vi "Number_To_String.vi"(1 "Number":dbl) -> (0 "String":string)   [LabVIEW 2011]
doc: "This VI will convert a number to a string without appending any unecessary zeros."
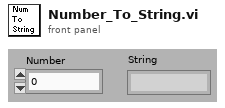
[diagram p1: front panel]
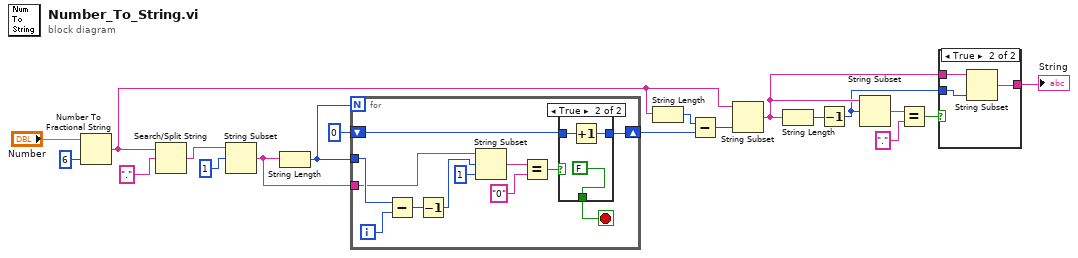
[diagram p0: block diagram]
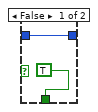
[diagram p3: hidden frame]
diagram:
  n1 = Number To Fractional String(number="Number", precision (6)=i16 6) -> (F-format string=w9:string)  [unwired: 2 out]
  n2 = Search/Split String(string=w9, search string/char (-)="." ("search string")) -> (match + rest of string=w12:string)  [unwired: 3 out]
  n3 = String Subset(string=w12, offset (0)=1) -> (substring=w13:string)  [unwired: 1 out]
  n4 = String Length(string=w13) -> (length=w15:i32)
  n5 = for {
    N: w15 -> [_]
    tunnel: w15 -> [w29]
    shift-right: [w22] -> w11
    shift-left: 0 -> [w21]
    tunnel: w13 -> [w27]
    i -> [w31]
    stop <- w20 stop-if-true
    n6 = Subtract(x=w29, y=w31) -> (x-y=w30:i32)
    n7 = Decrement(x=w30) -> (x-1=w25:i32)
    n8 = String Subset(string=w27, offset (0)=w25, length (rest)=1 ("length (rest)")) -> (substring=w26:string)
    n9 = Equal?(x=w26, y="0") -> (x = y?=w23:bool)
    n10 = case shown="True" w23 {
      tunnel: [w33 w36] -> w22
      tunnel: w21 -> [w33 w35]
      tunnel: [TRUE FALSE] -> w20
      frame False {
      }
      frame True {
        n11 = Increment(x=w35) -> (x+1=w36:i32)
      }
    }
  }
  n12 = String Length(string=w9) -> (length=w10:i32)
  n13 = Subtract(x=w10, y=w11) -> (x-y=w8:i32)
  n14 = String Subset(string=w9, length (rest)=w8) -> (substring=w2:string)  [unwired: 1 out]
  n15 = String Length(string=w2) -> (length=w7:i32)
  n16 = Decrement(x=w7) -> (x-1=w1:i32)
  n17 = String Subset(string=w2, offset (0)=w1) -> (substring=w6:string)  [unwired: 1 out]
  n18 = Equal?(x=w6, y=".") -> (x = y?=w4:bool)
  n19 = case shown="True" w4 {
    tunnel: [w37 w38] -> w3
    tunnel: w2 -> [w37 w40]
    tunnel: w1 -> [_ w39]
    frame False {
    }
    frame True {
      n20 = String Subset(string=w40, length (rest)=w39) -> (substring=w38:string)  [unwired: 1 out]
    }
  }
  "String" <- w3
